vi "Reset Dependencies.vi"(8 "error in (no error)":errorcluster, 11 "Device Ref in":T1 format="%.0x") -> (0 "error out":errorcluster, 3 "Dev Ref out":T1 format="%.0x")   [LabVIEW 2011, in "TDMS Custom Device.lvlib"]
uses:
  TDMS Custom Device.lvlib
  <vilib>/NI Veristand/Custom Device API/Custom Device Item Ref.ctl
  NationalInstruments.VeriStand.SystemStorage
  <vilib>/NI Veristand/Custom Device API/Custom Device API.lvlib
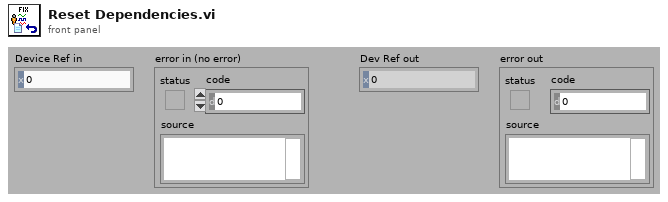
[diagram p1: front panel]
types:
  T1 = typedef "Custom Device API.lvlib/Custom Device Item Ref.ctl" = u64
  T2 = typedef "Custom Device API.lvlib/Custom Device Pointer.ctl" = refnum<k24>
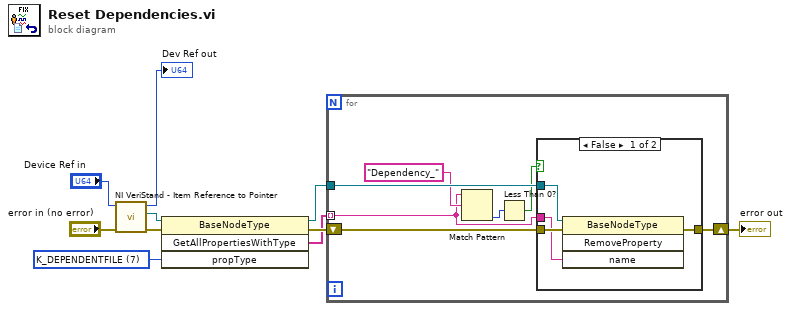
[diagram p0: block diagram]
diagram:
  w5 = 7 items=["K_STRING", "K_BOOL", "K_I32", "K_U32", "K_DOUBLE", "K_U64", "K_VARIANT", "K_DEPENDENTFILE", "K_DEPENDENTNODE", "K_DATASOURCENODE", "K_U16", "K_DBLARR", "K_U32ARR", "K_I32ARR", "K_STRINGARR", "K_DICTIONARY", "K_DICTIONARYARR", "K_BINARYSTRING"] ("propType")
  n1 = call <vilib>:"NI VeriStand - Item Reference to Pointer.vi"("error in (no error)"="error in (no error)", "Item Ref in"="Device Ref in") -> ("error out"=w4:errorcluster, "Node Pointer"=w6:T2, "Item Ref out"=→"Dev Ref out":T1)  [unwired: 6 in, 1 out]
  n2 = invoke class="BaseNodeType" method="GetAllPropertiesWithType"(reference=w6, error in=w4, "propType"=w5) -> (reference out=w2:T2, error out=w3:errorcluster, "GetAllPropertiesWithType"=w1:string[])  [unwired: 1 in, 1 out]
  n3 = for {
    shift-right: [w16] -> w10
    shift-left: w3 -> [w17]
    tunnel: w2 -> [w15]
    tunnel: w1 -> [w11] mode=indexing
    n4 = Match Pattern(string=w11, regular expression="Dependency_") -> (offset past match=w13:i32)  [unwired: 1 in, 3 out]
    n5 = Less Than 0?(x=w13) -> (x < 0?=w12:bool)
    n6 = case shown="False" w12 {
      tunnel: w17 -> [w21 w22]
      tunnel: [w20 w22] -> w16
      tunnel: w15 -> [w19 _]
      tunnel: w11 -> [w18 _]
      frame False {
        n7 = invoke class="BaseNodeType" method="RemoveProperty"(reference=w19, error in=w21, "name"=w18) -> (error out=w20:errorcluster)  [unwired: 1 in, 3 out]
      }
      frame True {
      }
    }
  }
  "error out" <- w10
